vi "Examples - ImgParams.vi"() -> ()   [LabVIEW 2013]
uses:
  xiLIB/xiCamLib/xiCam/PRM/IMG_FORMAT/IMG_DATA_FORMAT.ctl
panel:
  out "IMG_FORMAT":T1=enum."RAW16"
  out "DigitalInputLevel":i32
  out "Height":i32
  out "Width":i32
  out "GetBlackLevel":i32
  out "TimeStamp":dbl
  out "FrameNumber":i32
  out "DataFormat":i32
  in  "Stop":bool
  out "Image":T2(plugin-control)
  # "Use this button instead of Abort Execution button"
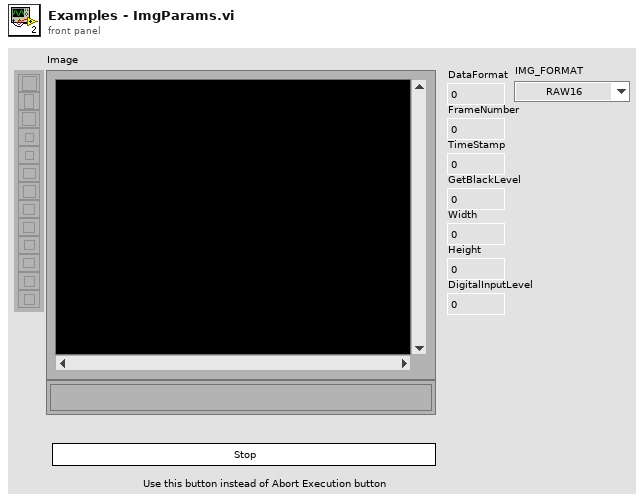
[diagram p1: front panel]
types:
  T1 = typedef "IMG_DATA_FORMAT.ctl" = enum16{"MONO8", "MONO16", "RGB24", "RGB32", "RGBPLANAR", "RAW8", "RAW16"}
  T2 = typedef "IMAQ Image.ctl" = refnum<image>
  T3 = typedef "xiImageMng - Attributes.ctl" = cluster{"WIDTH":i32, "HEIGHT":i32, "IMG_FORMAT":T1}
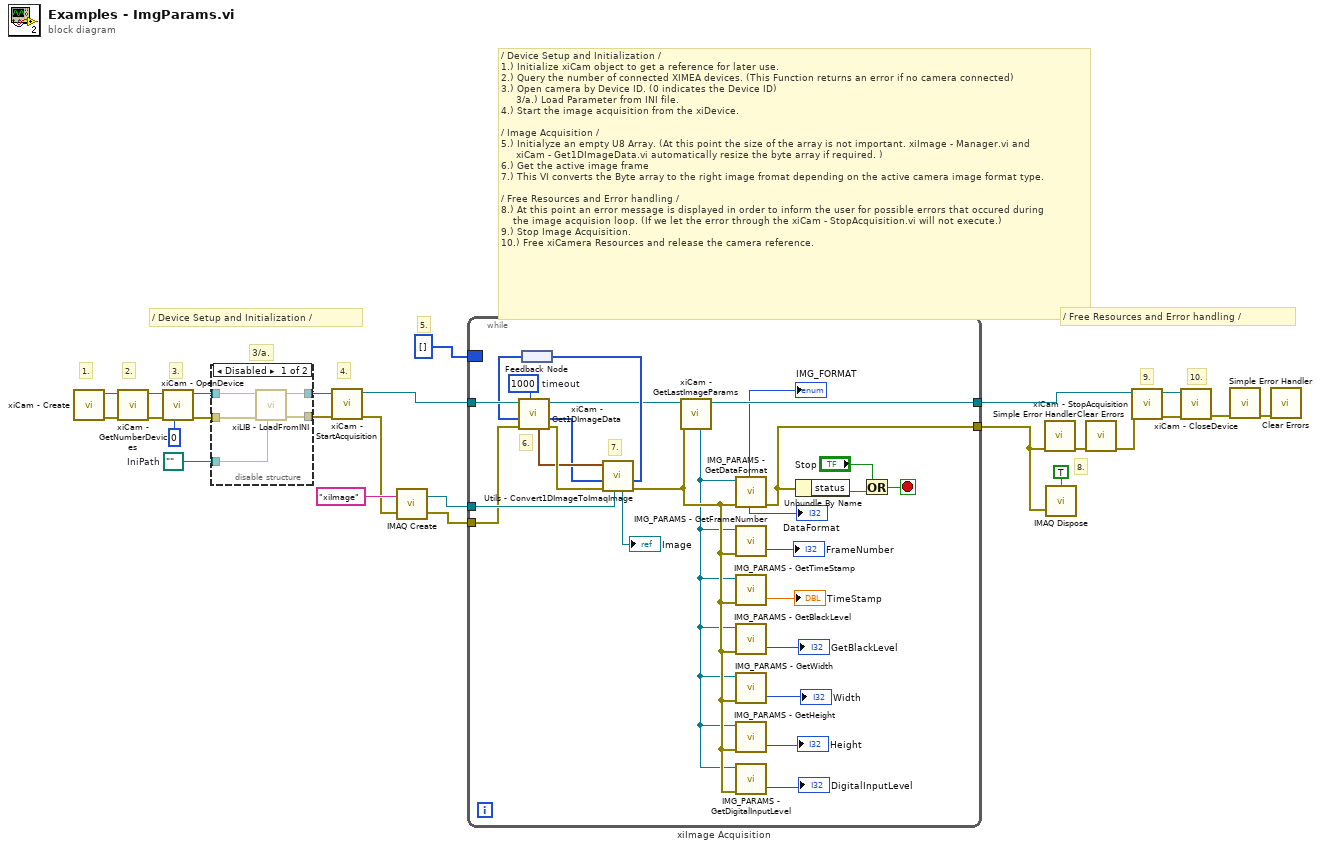
[diagram p0: block diagram]
diagram:
  w3 = path ""  # IniPath
  # "3/a."
  # "/ Free Resources and Error handling /"
  # "/ Device Setup and Initialization /"
  # "9."
  # "10."
  # "8."
  # "5."
  # "/ Device Setup and Initialization /\n1.) Initialize xiCam object to get a reference for later use.\n2.) Query the number of connected XIMEA devices. (This Function returns an error if no camera connected)\n3.) Open camera by Device ID. (0 indicates the Device ID)\n     3/a.) Load Parameter from INI file. \n4.) Start the image acquisition from the xiDevice.\n\n/ Image Acquisition /\n5.) Initialyze an empty U8 Array. (At this point the size of the array is not important. xiImage - Manager.vi and\n     xiCam - Get1DImageData.vi automatically resize the byte array if required. )\n6.) Get the active image frame\n7.) This VI converts the Byte array to the right image fromat depending on the active camera image format type.\n\n/ Free Resources and Error handling /\n8.) At this point an error message is displayed in order to inform the user for possible errors that occured during\n    the image acquision loop. (If we let the error through the xiCam - StopAcquisition.vi will not execute.)\n9.) Stop Image Acquisition.\n10.) Free xiCamera Resources and release the camera reference."
  # "4."
  # "3."
  # "2."
  # "1."
  n1 = call "xiCam - Create.vi"() -> ("error out"=w24:errorcluster, "new xiCam"=w25:refnum<k24>)  [unwired: 10 in]
  n2 = call "xiCam - GetNumberDevices.vi"("error in (no error)"=w24, "xiCam In"=w25) -> ("error out"=w22:errorcluster, "xiCam Out"=w23:refnum<k24>)  [unwired: 7 in, 1 out]
  n3 = call "xiCam - OpenDevice.vi"("DevID"=0, "error in (no error)"=w22, "xiCam In"=w23) -> ("error out"=w4:errorcluster, "xiCam Out"=w7:refnum<k24>)  [unwired: 7 in]
  n4 = disable-structure shown="Disabled" {
    disable-tunnel: w7 -> [w30 w32]
    disable-tunnel: [w29 w32] -> w6
    disable-tunnel: [w28 w31] -> w5
    disable-tunnel: w4 -> [w27 w31]
    disable-tunnel: w3 -> [w26 _]
    frame Disabled {
      n5 = call "xiLIB - LoadFromINI.vi"("IniPath"=w26, "Error In"=w27, "xiCam In"=w30) -> ("Error Out"=w28:errorcluster, "xiCam Out"=w29:refnum<k24>)  [unwired: 7 in]
    }
    frame Enabled {
    }
  }
  n6 = call "xiCam - StartAcquisition.vi"("error in (no error)"=w5, "xiCam In"=w6) -> ("error out"=w9:errorcluster, "xiCam Out"=w20:refnum<k24>)  [unwired: 8 in]
  n7 = call "IMAQ Create"("Image Name"="xiImage", "error in (no error)"=w9) -> ("New Image"=w10:T2, "error out"=w8:errorcluster)  [unwired: 3 in]
  n8 = while "xiImage Acquisition" {
    tunnel: w20 -> [w58]
    border: u8[] [] ("1DImageData Out") -> [_]
    tunnel: [w43] -> w2
    tunnel: [w44] -> w18
    tunnel: w10 -> [w48]
    tunnel: w8 -> [w47]
    stop <- w49 stop-if-true
    w56 = 1000  # timeout
    # "7."
    # "6."
    n9 = feedback #1() -> (w57:u8[])
    n10 = call "xiCam - Get1DImageData.vi"("timeout"=w56, "error in (no error)"=w47, "1DImageData In"=w57, "xiCam In"=w58) -> ("error out"=w55:errorcluster, "1DImageData Out"=w53:u8[], "xiCam Out"=w45:refnum<k24>, "Image Properites"=w54:T3)  [unwired: 4 in]
    n11 = call "Utils - Convert1DImageToImaqImage.vi"("Image In"=w48, "error in (no error)"=w55, "1DImageData In"=w53, "Image Properties In"=w54) -> ("error out"=w38:errorcluster, "1DImageData Out"=w52:u8[], "Image Out"=→"Image":T2)  [unwired: 5 in]
    n12 = feedback-in #1(w52) -> ()
    n13 = call "xiCam - GetLastImageParams.vi"("error in (no error)"=w38, "xiCam In"=w45) -> ("xiCam Out"=w44:refnum<k24>, "GetLastImageParams"=w34:refnum<k24>)  [unwired: 7 in, 1 out]
    n14 = call "IMG_PARAMS - GetDataFormat.vi"("error in (no error)"=w38, "xiApi.NET.ImgParams"=w34) -> ("error out"=w43:errorcluster, "DataFormat"=→"DataFormat":i32, "IMG_FORMAT"=→"IMG_FORMAT":T1)  [unwired: 6 in, 1 out]
    n15 = call "IMG_PARAMS - GetFrameNumber.vi"("error in (no error)"=w38, "xiApi.NET.ImgParams"=w34) -> ("FrameNumber"=→"FrameNumber":i32)  [unwired: 7 in, 2 out]
    n16 = call "IMG_PARAMS - GetTimeStamp.vi"("error in (no error)"=w38, "xiApi.NET.ImgParams"=w34) -> ("TimeStamp"=→"TimeStamp":dbl)  [unwired: 7 in, 2 out]
    n17 = call "IMG_PARAMS - GetBlackLevel.vi"("error in (no error)"=w38, "xiApi.NET.ImgParams"=w34) -> ("GetBlackLevel"=→"GetBlackLevel":i32)  [unwired: 7 in, 2 out]
    n18 = call "IMG_PARAMS - GetWidth.vi"("error in (no error)"=w38, "xiApi.NET.ImgParams"=w34) -> ("Width"=→"Width":i32)  [unwired: 7 in, 2 out]
    n19 = call "IMG_PARAMS - GetHeight.vi"("error in (no error)"=w38, "xiApi.NET.ImgParams"=w34) -> ("Height"=→"Height":i32)  [unwired: 7 in, 2 out]
    n20 = call "IMG_PARAMS - GetDigitalInputLevel.vi"("error in (no error)"=w38, "xiApi.NET.ImgParams"=w34) -> ("DigitalInputLevel"=→"DigitalInputLevel":i32)  [unwired: 7 in, 2 out]
    n21 = Unbundle By Name(w43) -> ("status"=w51:bool)
    n22 = Or(x="Stop", y=w51) -> (x .or. y?=w49:bool)
  }
  n23 = call <vilib>:"Simple Error Handler.vi"("error in (no error)"=w2) -> ("error out"=w17:errorcluster)  [unwired: 4 in, 4 out]
  n24 = call "IMAQ Dispose"("All Images? (No)"=TRUE, "error in (no error)"=w2) -> ()  [unwired: 4 in, 1 out]
  n25 = call <vilib>:"Clear Errors.vi"("error in (no error)"=w17) -> ("error out"=w16:errorcluster)  [unwired: 6 in]
  n26 = call "xiCam - StopAcquisition.vi"("error in (no error)"=w16, "xiCam In"=w18) -> ("error out"=w14:errorcluster, "xiCam Out"=w15:refnum<k24>)  [unwired: 8 in]
  n27 = call "xiCam - CloseDevice.vi"("error in (no error)"=w14, "xiCam In"=w15) -> ("error out"=w12:errorcluster)  [unwired: 9 in]
  n28 = call <vilib>:"Simple Error Handler.vi"("error in (no error)"=w12) -> ("error out"=w13:errorcluster)  [unwired: 4 in, 4 out]
  n29 = call <vilib>:"Clear Errors.vi"("error in (no error)"=w13) -> ()  [unwired: 6 in, 1 out]
